vi "Load X minus Previous Delta.vi"(7 "Reinit":bool, 8 "error in (no error)":errorcluster, 10 "X":dbl, 11 "Stats_DBL_CIF_U in":refnum<class "Stats_DBL_CIF_U.lvclass">) -> (0 "error out":errorcluster, 3 "Stats_DBL_CIF_U out":refnum<class "Stats_DBL_CIF_U.lvclass">)   [LabVIEW 2021, in "Stats_CIF_U.lvlib" / "Stats_DBL_CIF_U.lvclass"]
doc: "Load a new data value into the statistics class. The new value will be calculated by subracting the new X value from the last value added to the class. This VI is useful for cyclic timing where timestamps are provided as input X."
uses:
  Stats_DBL_CIF_U.lvclass
  Stats_DBL_CIF_U.lvclass/Stats_DBL_CIF_U.ctl
  dfabcf33-0dbc-4041-80a5-3dc0c86d2989.vi
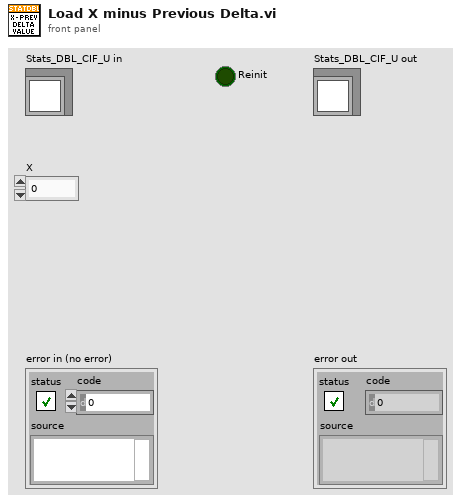
[diagram p1: front panel]
types:
  T1 = typedef "Stats_CIF_U.lvlib/DBL Stat Data.ctl" = cluster{"Last Value":dbl, "Max":dbl, "Min":dbl, "Common ":T2}
  T2 = typedef "Stats_CIF_U.lvlib/Common Stat Data.ctl" = cluster{"Iteration":u32, "Max History":i32, "Average":dbl}
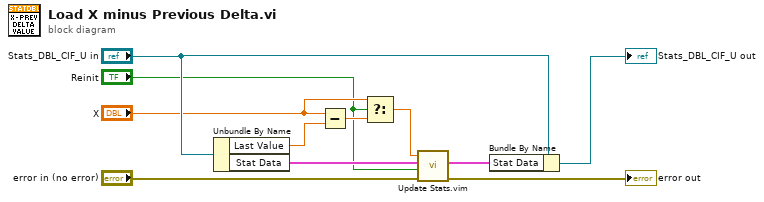
[diagram p0: block diagram]
diagram:
  n1 = Unbundle By Name("Stats_DBL_CIF_U in") -> ("Last Value"=w6:dbl, "Stat Data"=w5:T1)
  n2 = Subtract(x="X", y=w6) -> (x-y=w4:dbl)
  n3 = Select(t="X", s="Reinit", f=w4) -> (s? t:f=w2:dbl)
  n4 = call "Update Stats.vim"("error in"="error in (no error)", "Load Value Only"="Reinit", "Stat Data In"=w5, "New Value"=w2) -> ("error out"=→"error out":errorcluster, "Stat Data Out"=w10:T1)  [unwired: 6 in]
  n5 = Bundle By Name(cluster="Stats_DBL_CIF_U in", "Stat Data"=w10) -> (→"Stats_DBL_CIF_U out":refnum<class "Stats_DBL_CIF_U.lvclass">)
